vi "dac_test_pattern.vi"() -> ()   [LabVIEW 2014]
uses:
  <vilib>/measure/NI_MABase.lvlib
panel:
  in  "Output file":path=path "C:/Data/foo.bin"
  out "transposed array":i32[][](array[numeric])
  out "output array":i32[](array[numeric])
  in  "signal type":T1(ring)=enum."Triangle Wave"
  in  "sampling info":cluster{"Fs":dbl, "#s":dbl}={"Fs"=48828.0, "#s"=16384.0} {"Fs" format="%.2p"}
  out "Waveform Graph":waveform(dbl)[](graph)
  in  "Phase shift (degrees)":dbl=10.0
  in  "Frequency  (Hz)":dbl=48.83
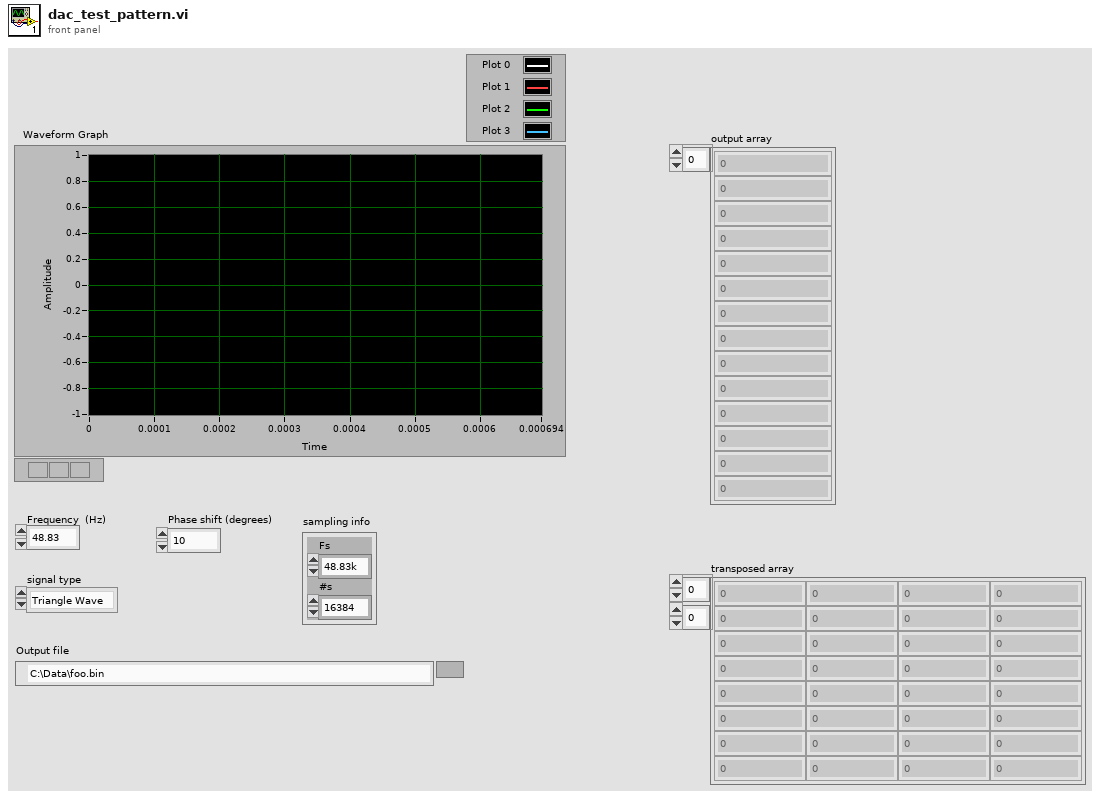
[diagram p1: front panel]
types:
  T1 = enum16{"Sine Wave", "Triangle Wave", "Square Wave", "Sawtooth Wave"}
  T2 = enum16{"big-endian, network order", "native, host order", "little-endian"}
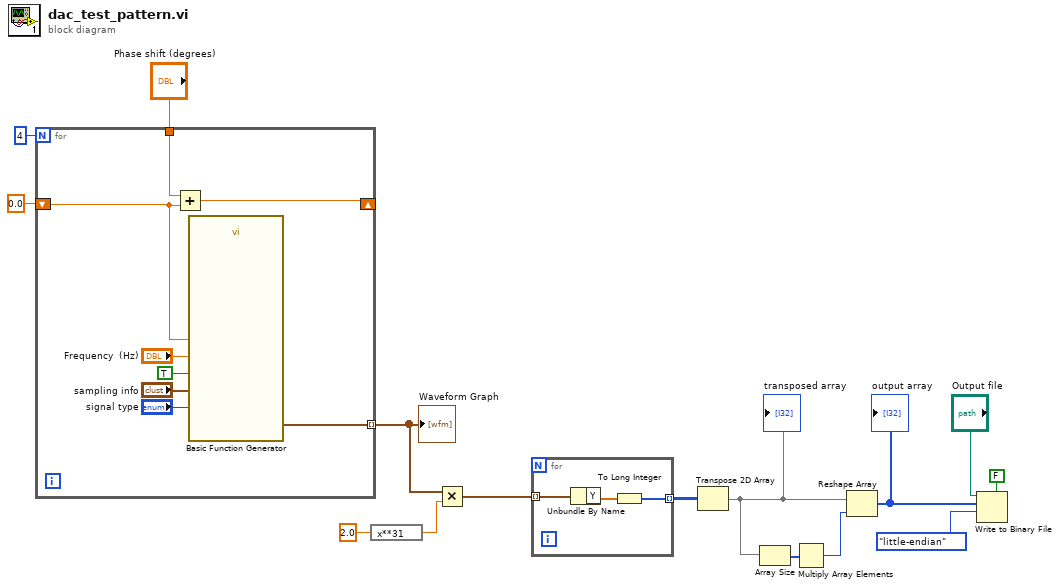
[diagram p0: block diagram]
diagram:
  n1 = for {
    N: 4 -> [_]
    shift-right: [w22] -> _
    shift-left: 0.0 ("Phase shift (degrees)") -> [w16]
    tunnel: "Phase shift (degrees)" -> [w21]
    tunnel: [w17] -> w12 mode=indexing
    n2 = Add(x=w21, y=w16) -> (x+y=w22:dbl)
    n3 = call <vilib>:"Basic Function Generator.vi"("reset signal"=TRUE, "sampling info"="sampling info", "signal type"="signal type", "phase"=w16, "frequency"="Frequency  (Hz)") -> ("signal out"=w17:waveform(dbl))  [unwired: 4 in, 2 out]
  }
  "Waveform Graph" <- w12
  n4 = expression code="x**31"(2.0 ("x+y")) -> (w10:dbl)
  n5 = Multiply(x=w12, y=w10) -> (x*y=w9:waveform(dbl)[])
  n6 = for {
    tunnel: w9 -> [w26] mode=indexing
    tunnel: [w24] -> w8 mode=indexing
    n7 = Unbundle By Name(w26) -> ("Y"=w25:dbl[])
    n8 = To Long Integer(number=w25) -> (32bit integer=w24:i32[])
  }
  n9 = Transpose 2D Array(2D array=w8) -> (transposed array=w4:i32[][])
  "transposed array" <- w4
  n10 = Array Size(array=w4) -> (size(s)=w7:i32[])
  n11 = Multiply Array Elements(1:w7) -> (0:w6:i32)
  n12 = Reshape Array(w4, w6) -> (w3:i32[])
  "output array" <- w3
  n13 = Write to Binary File(file (use dialog)="Output file", data=w3, 5:FALSE ("prepend array or string size? (T)"), 9:T2."little-endian" ("byte order (0:big-endian, network order)")) -> ()  [unwired: 2 in, 3 out]
